vi "Hide Window.vi"(0 "Py Doc in":refnum<class "Py Doc.lvclass">, 11 "error in (no error)":errorcluster) -> (4 "Py Doc out":refnum<class "Py Doc.lvclass">, 15 "error out":errorcluster)   [LabVIEW 2016, in "Py Doc.lvclass"]
uses:
  Py Doc.lvclass
  D:/git/LabVIEW-MDI/source code/Document/Document.lvclass
  Document.lvclass/Document.ctl
  Py Doc.lvclass/Py Doc.ctl
  user32.dll
  Document.lvclass
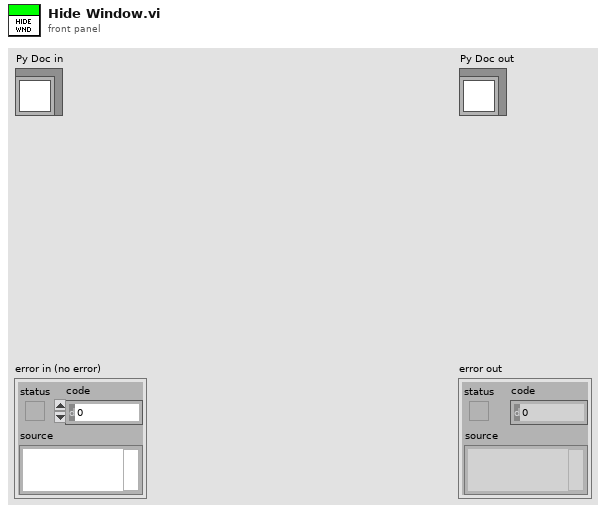
[diagram p1: front panel]
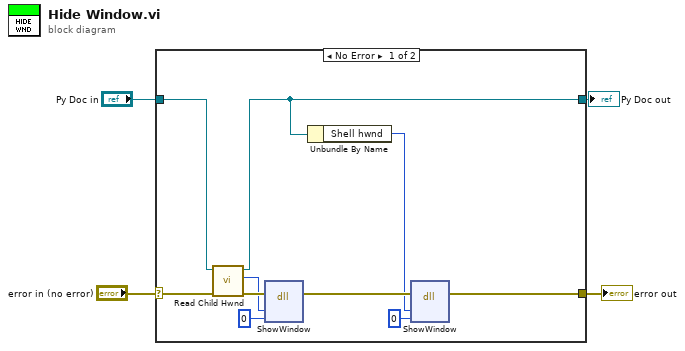
[diagram p0: block diagram]
diagram:
  n1 = case shown="No Error" "error in (no error)" {
    selector: "error in (no error)" -> [w11 w15]
    tunnel: [w7 w15] -> w3
    tunnel: "Py Doc in" -> [w10 w16]
    tunnel: [w9 w16] -> w1
    frame No Error {
      n2 = call "Read Child Hwnd.vi"("error in (no error)"=w11, "Document in"=w10) -> ("error out"=w13:errorcluster, "Child Hwnd"=w12:u32, "Document out"=w9:refnum<class "Py Doc.lvclass">)  [unwired: 7 in]
      n3 = dll-call lib="user32.dll" fn="ShowWindow"(error in=w13, "hwnd"=w12, "nCmdShow"=u32 0) -> (error out=w8:errorcluster)  [unwired: 5 in, 1 out]
      n4 = Unbundle By Name(w9) -> ("Shell hwnd"=w5:u32)
      n5 = dll-call lib="user32.dll" fn="ShowWindow"(error in=w8, "hwnd"=w5, "nCmdShow"=u32 0) -> (error out=w7:errorcluster)  [unwired: 5 in, 1 out]
    }
    frame Error {
    }
  }
  "error out" <- w3
  "Py Doc out" <- w1
